vi "Destroy.vi"(8 "error in (no error)":errorcluster, 11 "JKI SMO in":refnum<class "JKI SMO.lvclass">) -> (0 "error out":errorcluster)   [LabVIEW 2013, in "JKI SMO.lvclass"]
doc: "Destructor\n\nNote 01: This method is overridable by descendant\nNote 02: When overridden, Call Parent Method is required\n\n---------------------------------------------------------------\nJKI State Machine Objects™\nhttp://jki.net/state-machine-objects/\nCopyright (C) 2005-2015, JKI <info@jki.net>\nALL RIGHTS RESERVED"
uses:
  JKI SMO.lvclass
  JKI SMO.lvclass/JKI SMO.ctl
panel:
  # "For instructions on how to use the JKI State Machine Objects, examples and video tutorials, visit:\nhttp://jki.net/state-machine-objects/\n\nJKI State Machine Objects™\nhttp://jki.net/state-machine-objects/\nCopyright (C) 2005-2015, JKI <info@jki.net>\nALL RIGHTS RESERVED"
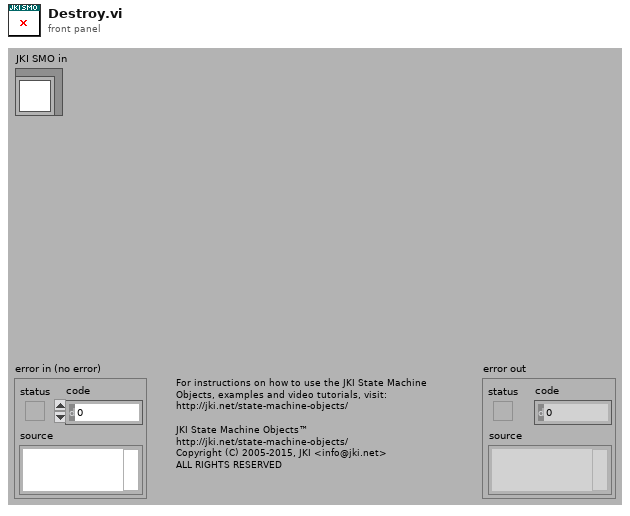
[diagram p1: front panel]
types:
  T1 = typedef "pSubSystem.lvclass/pSubSystem.PrivateData--Cluster.ctl" = cluster{"Processes Clone VI Ref [ ]":refnum<vi>[], "Processes Clone Name [ ]":string[], "Process Sync RendezVous":T2, "Protected Events":T3}
  T2 = typedef "Rendezvous RefNum" = refnum<k1>
  T3 = typedef "pSubSystem.lvclass/pSubSystem.ProtectedEvents--Cluster.ctl" = cluster{"StopProcesses":refnum<user-event>, "AbortProcesses":refnum<user-event>}
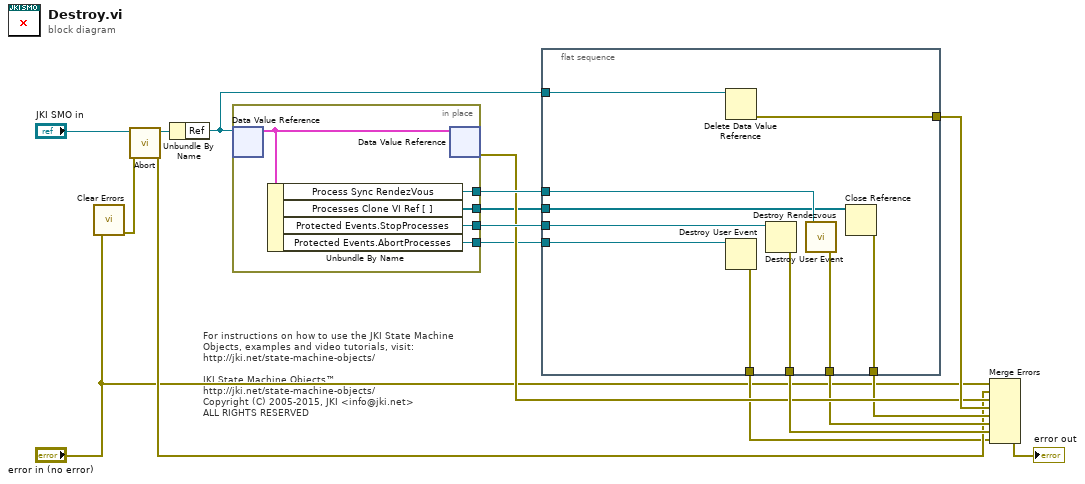
[diagram p0: block diagram]
diagram:
  # "For instructions on how to use the JKI State Machine Objects, examples and video tutorials, visit:\nhttp://jki.net/state-machine-objects/\n\nJKI State Machine Objects™\nhttp://jki.net/state-machine-objects/\nCopyright (C) 2005-2015, JKI <info@jki.net>\nALL RIGHTS RESERVED"
  n1 = call <vilib>:"Clear Errors.vi"("error in (no error)"="error in (no error)") -> ("error out"=w1:errorcluster)  [unwired: 6 in]
  n2 = call "Abort.vi"("error in (no error)"=w1, "JKI SMO in"="JKI SMO in") -> ("error out"=w5:errorcluster, "JKI SMO out"=w6:refnum<class "JKI SMO.lvclass">)  [unwired: 8 in]
  n3 = Unbundle By Name(w6) -> ("Ref"=w15:refnum<data-value>)
  n4 = in-place {
    in-place-border: [w21] -> w17
    in-place-border: [w20] -> w13
    in-place-border: [w19] -> w10
    in-place-border: [w18] -> w4
    n5 = in-place-dvr #1(w15) -> (w22:T1)  [unwired: 1 out]
    n6 = Unbundle By Name(w22) -> ("Process Sync RendezVous"=w20:T2, "Processes Clone VI Ref [ ]"=w19:refnum<vi>[], "Protected Events.StopProcesses"=w21:refnum<user-event>, "Protected Events.AbortProcesses"=w18:refnum<user-event>)
    n7 = in-place-dvr #1(w22) -> (w11:errorcluster)  [unwired: 1 out]
  }
  n8 = flat-sequence {
    tunnel: w17 -> [w25]
    tunnel: w15 -> [w32]
    tunnel: [w31] -> w14
    tunnel: w13 -> [w30]
    tunnel: [w29] -> w12
    tunnel: w10 -> [w27]
    tunnel: [w28] -> w9
    tunnel: [w26] -> w8
    tunnel: w4 -> [w24]
    tunnel: [w23] -> w3
    frame #0 {
      n9 = Delete Data Value Reference(data value reference=w32) -> (error out=w31:errorcluster)  [unwired: 1 in, 1 out]
      n10 = Destroy User Event(user event=w24) -> (error out=w23:errorcluster)  [unwired: 1 in]
      n11 = Destroy User Event(user event=w25) -> (error out=w29:errorcluster)  [unwired: 1 in]
      n12 = call <vilib>:"Destroy Rendezvous.vi"("rendezvous"=w30) -> ("error out"=w28:errorcluster)  [unwired: 5 in, 1 out]
      n13 = Close Reference(reference=w27) -> (error out=w26:errorcluster)  [unwired: 1 in]
    }
  }
  n14 = Merge Errors("error in (no error)", w5, w11, w14, w8, w9, w12, w3) -> (→"error out":errorcluster)
